vi "Cannon Get.vi"() -> ()   [LabVIEW 2013]
uses:
  <vilib>/Rock Robotics/WPI/Solenoid/WPI_SolenoidValue.ctl
  Cannon Global Data.vi
panel:
  in  "Cannon":dbl
  in  "Solenoid":T1
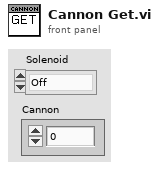
[diagram p1: front panel]
types:
  T1 = typedef "WPI_SolenoidValue.ctl" = enum16{"Off", "On", "Forward", "Reverse"}
  T2 = cluster{"Motor":dbl, "Solenoid":T1, "BallInMS":bool, "ClutchMS":bool, "Potentiometer":dbl}
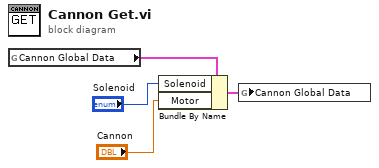
[diagram p0: block diagram]
diagram:
  n1 = global read "Cannon Global Data.vi" "Cannon Global Data"() -> (w4:T2)
  n2 = Bundle By Name(cluster=w4, "Solenoid"="Solenoid", "Motor"="Cannon") -> (w2:T2)
  n3 = global write "Cannon Global Data.vi" "Cannon Global Data"(w2) -> ()
